vi "Write #slam dunks.vi"(8 "error in (no error)":errorcluster, 10 "#slam dunks":u64, 11 "Shaquille O'Neal in":refnum<class "Shaquille O'Neal.lvclass">) -> (0 "error out":errorcluster, 3 "Shaquille O'Neal out":refnum<class "Shaquille O'Neal.lvclass">)   [LabVIEW 2019, in "Shaquille O'Neal.lvclass"]
uses:
  Shaquille O'Neal.lvclass
  Shaquille O'Neal.lvclass/Shaquille O'Neal.ctl
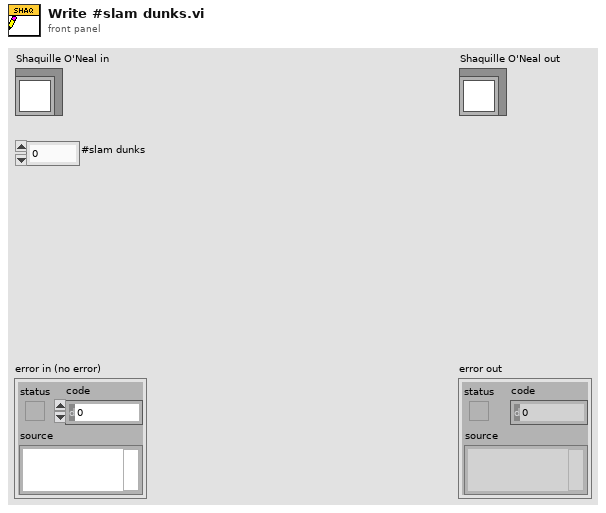
[diagram p1: front panel]
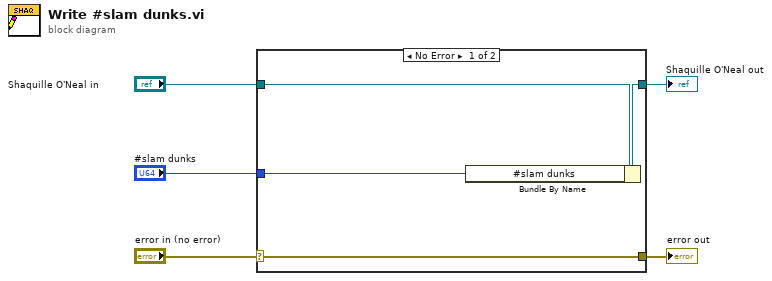
[diagram p0: block diagram]
diagram:
  n1 = case shown="No Error" "error in (no error)" {
    selector: "error in (no error)" -> [w9 w10]
    tunnel: [w9 w10] -> w4
    tunnel: [w7 w11] -> w2
    tunnel: "Shaquille O'Neal in" -> [w8 w11]
    tunnel: "#slam dunks" -> [w6 _]
    frame No Error {
      n2 = Bundle By Name(cluster=w8, "#slam dunks"=w6) -> (w7:refnum<class "Shaquille O'Neal.lvclass">)
    }
    frame Error {
    }
  }
  "error out" <- w4
  "Shaquille O'Neal out" <- w2
